vi "Create.vi"(11 "API out 2":refnum<class "API.lvclass">) -> (3 "API out":refnum<class "API.lvclass">)   [LabVIEW 2024, in "API.lvclass"]
uses:
  API.lvclass
  Message.ctl
  API.lvclass/API.ctl
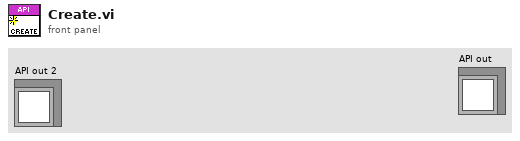
[diagram p1: front panel]
types:
  T1 = typedef "API.lvclass/Message.ctl" = cluster{"Name":string, "Data":variant}
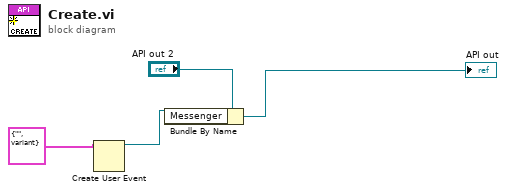
[diagram p0: block diagram]
diagram:
  n1 = Create User Event(user event datatype=T1 {"Name"="", "Data"=variant} ("Message")) -> (user event=w3:refnum<user-event>)  [unwired: 1 in, 1 out]
  n2 = Bundle By Name(cluster="API out 2", "Messenger"=w3) -> (→"API out":refnum<class "API.lvclass">)
